vi "Read Customer Name.vi"(11 "Beverage in":refnum<class "Beverage.lvclass">) -> (2 "Customer Name":string)   [LabVIEW 2013, in "Beverage.lvclass"]
uses:
  Beverage.lvclass
  Beverage.lvclass/Beverage.ctl
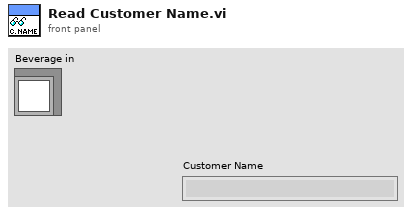
[diagram p1: front panel]
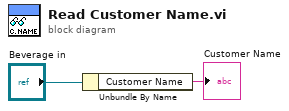
[diagram p0: block diagram]
diagram:
  n1 = Unbundle By Name("Beverage in") -> ("Customer Name"=→"Customer Name":string)
